vi "Toggle.vi"(6 "Reset":bool, 8 "Initial":bool, 11 "Toggle":bool) -> (3 "BoolOut":bool)   [LabVIEW 2012]
doc: "Toggles a internal boolean value if the boolean Toggle is true, and outputs the internal boolean value that was/was not toggled. If Initial is wired, the internal boolean value is instantiated to Initial.s"
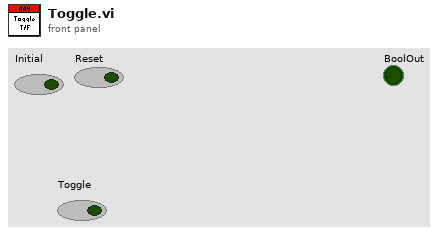
[diagram p1: front panel]
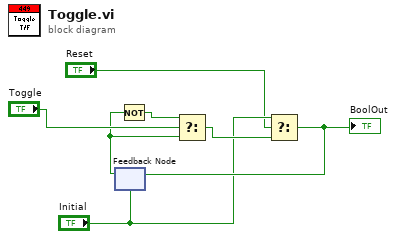
[diagram p0: block diagram]
diagram:
  n1 = feedback #1("Initial") -> (w5:bool)
  n2 = Not(x=w5) -> (.not. x?=w6:bool)
  n3 = Select(t=w6, s="Toggle", f=w5) -> (s? t:f=w3:bool)
  n4 = Select(t="Initial", s="Reset", f=w3) -> (s? t:f=w4:bool)
  "BoolOut" <- w4
  n5 = feedback-in #1(w4) -> ()
